vi "Wheel(2).vi"() -> ()   [LabVIEW 2020]
uses:
  <vilib>/DAQmx/read.llb/DAQmx Read (Counter DBL 1Chan 1Samp).vi
  <vilib>/DAQmx/create/channels.llb/DAQmx Create Channel (CI-Position-Angular Encoder).vi
  Shared/Experiment/ExperimentGlobals.vi
  <vilib>/Utility/file.llb/Write Delimited Spreadsheet (string).vi
  Shared/ModuleCrosstalk/Crosstalk.vi
  <vilib>/DAQmx/miscellaneous.llb/DAQmx Fill In Error Info.vi
  <vilib>/Utility/file.llb/Write Delimited Spreadsheet (DBL).vi
panel:
  out "Numeric":i32
  out "Speed av. 1s(cm/s) 2":dbl
  out "Output file":path
  out "Speed (cm/s)":dbl
  out "Counter task":refnum<k21>
  out "Aquiering":bool
  out "Distance (m)":dbl
  out "Angle (deg)":dbl
  out "Motion plot":dbl(graph)
  out "Recording":bool
  # "Mouse Wheel"
  # "Wires (left-right) : black-empty-green-orange-yellow"
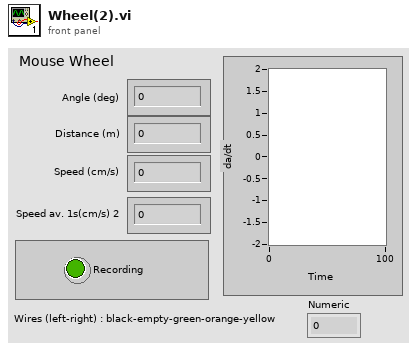
[diagram p1: front panel]
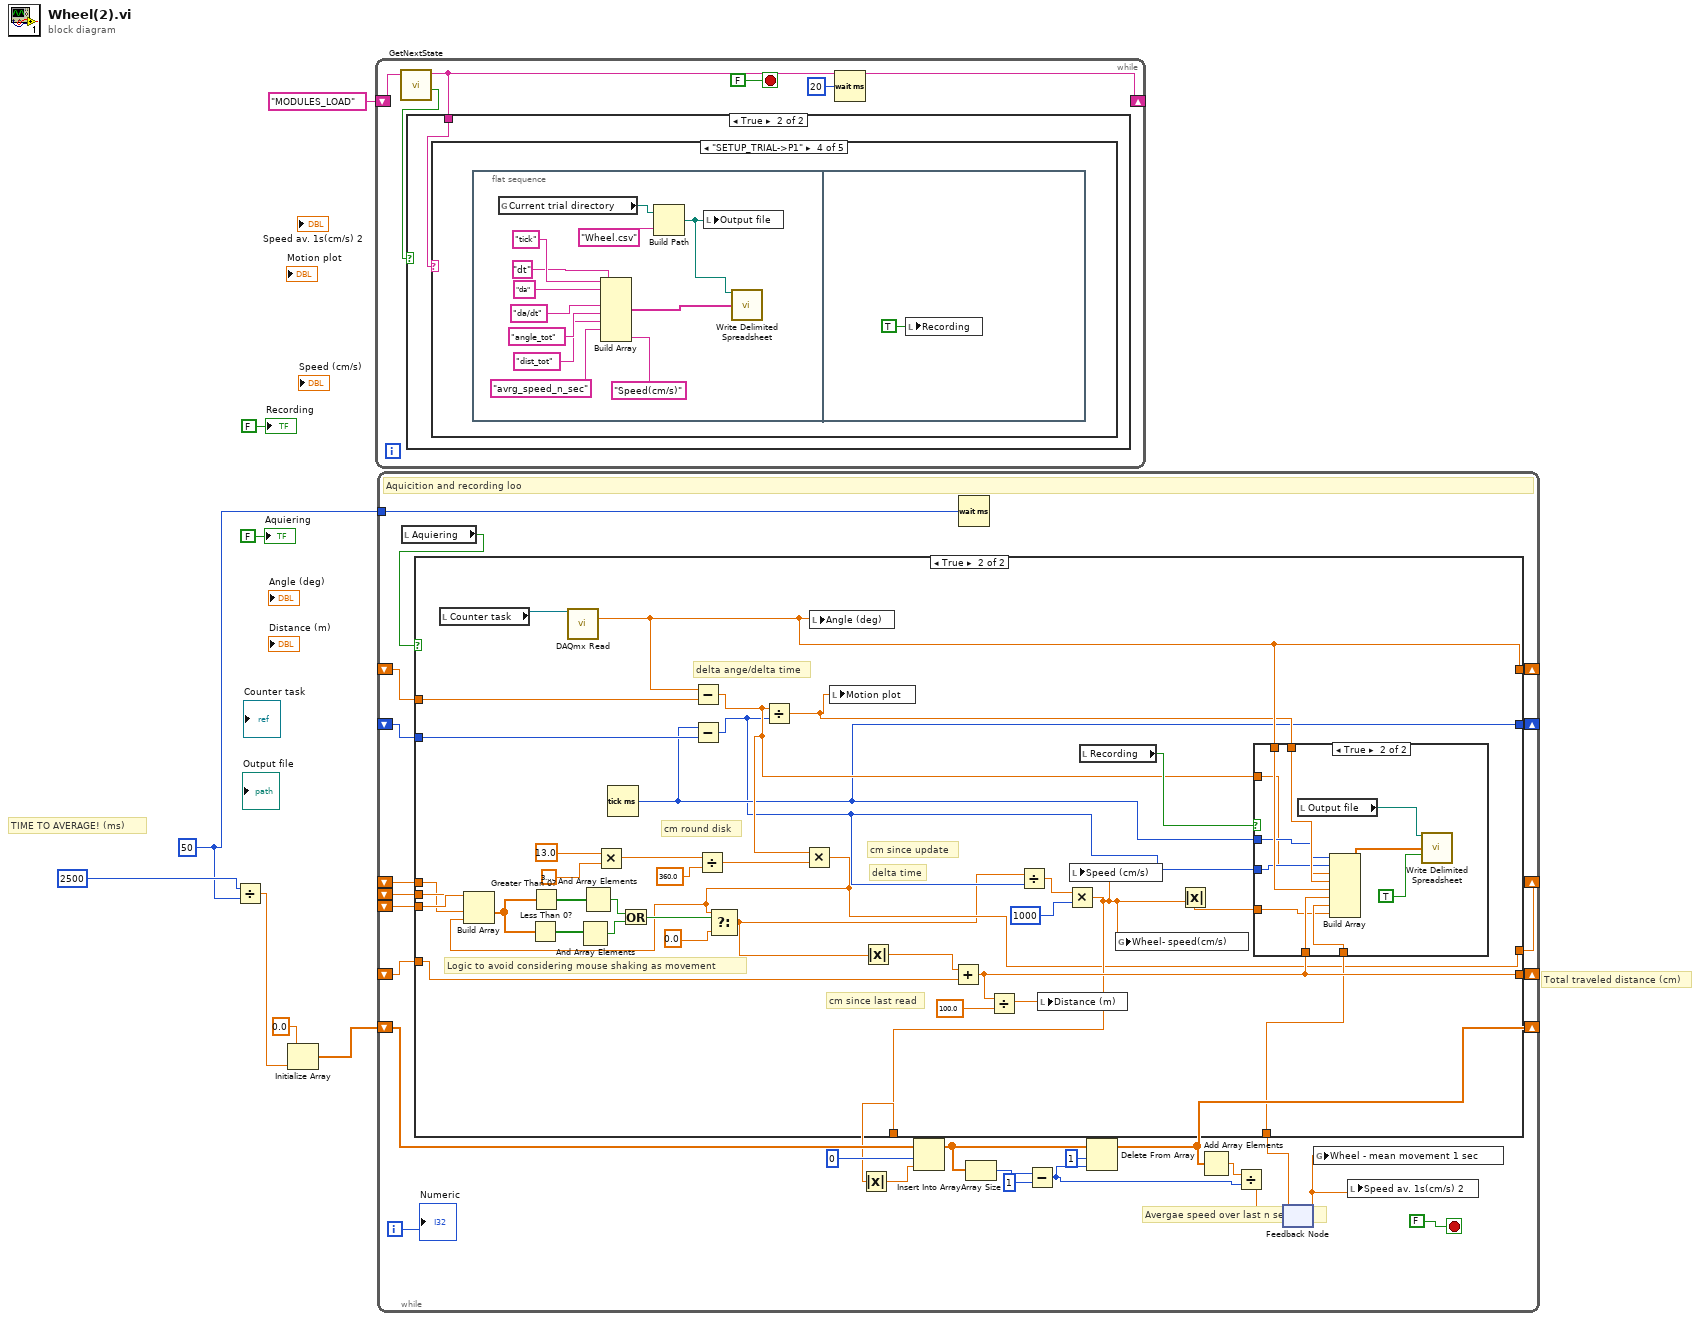
[diagram p0: block diagram]
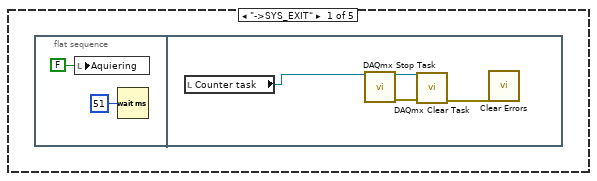
[diagram p5: hidden frame]
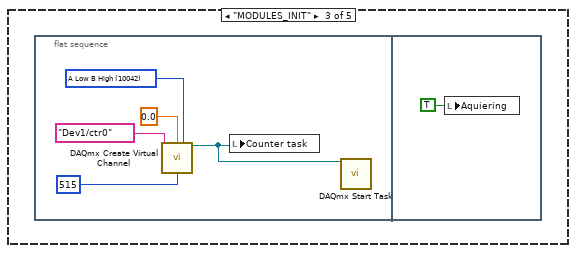
[diagram p7: hidden frame]
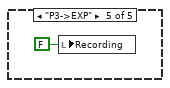
[diagram p8: hidden frame]
diagram:
  w4 = 50
  # "TIME TO AVERAGE! (ms)"
  # "Total traveled distance (cm)"
  n1 = Divide(x=2500, y=w4) -> (x/y=w3:dbl)
  n2 = Initialize Array(0.0, w3) -> (w1:dbl[])
  n3 = while {
    shift-right: [w9] -> _
    shift-left: "MODULES_LOAD" ("Next state") -> [w11]
    stop <- FALSE stop-if-true
    n4 = call "GetNextState.vi"("Current state"=w11) -> ("State has changed?"=w10:bool, "Next state"=w9:string)  [unwired: 9 in]
    n5 = case shown="True" w10 {
      tunnel: w9 -> [_ w14]
      frame False {
      }
      frame True {
        n6 = case shown="\"SETUP_TRIAL->P1\"" w14 {
          frame "->SYS_EXIT" {
            n7 = flat-sequence {
              frame #0 {
                n8 = local write "Aquiering"(FALSE ("Aquiering")) -> ()
                n9 = Wait (ms)(milliseconds to wait=u32 51) -> ()  [unwired: 1 out]
              }
              frame #1 {
                n10 = local read "Counter task"() -> (w17:refnum<k21>)
                n11 = call <vilib>:"DAQmx Stop Task.vi"("task/channels in"=w17) -> ("task out"=w18:refnum<k21>, "error out"=w19:errorcluster)  [unwired: 13 in]
                n12 = call <vilib>:"DAQmx Clear Task.vi"("task in"=w18, "error in"=w19) -> ("error out"=w20:errorcluster)  [unwired: 13 in]
                n13 = call <vilib>:"Clear Errors.vi"("error in (no error)"=w20) -> ()  [unwired: 5 in, 2 out]
              }
            }
          }
          frame Default {
          }
          frame "MODULES_INIT" {
            n14 = flat-sequence {
              frame #0 {
                w21 = 10042 items=["A High B High"=10040, "A High B Low"=10041, "A Low B High"=10042, "A Low B Low"=10043] ("z index phase")
                n15 = call-poly <vilib>:"DAQmx Create Virtual Channel.vi"("z index value"=0.0, "z index phase"=w21, "counter"=tag "Dev1/ctr0", "pulses per revolution"=u32 515) -> ("task out"=w23:refnum<k21>)  [unwired: 10 in, 1 out]
                n16 = local write "Counter task"(w23) -> ()
                n17 = call <vilib>:"DAQmx Start Task.vi"("task/channels in"=w23) -> ()  [unwired: 13 in, 2 out]
              }
              frame #1 {
                n18 = local write "Aquiering"(TRUE ("Aquiering")) -> ()
              }
            }
          }
          frame "SETUP_TRIAL->P1" {
            n19 = flat-sequence {
              frame #0 {
                n20 = global read "ExperimentGlobals.vi" "Current trial directory"() -> (w38:path)
                n21 = Build Array("tick", "dt" ("element"), "da" ("element"), "da/dt" ("element"), "angle_tot" ("element"), "dist_tot" ("element"), "avrg_speed_n_sec" ("element"), "Speed(cm/s)" ("element")) -> (w35:string[])
                n22 = Build Path(base path=w38, name or relative path="Wheel.csv") -> (appended path=w36:path)
                n23 = local write "Output file"(w36) -> ()
                n24 = call-poly <vilib>:"Write Delimited Spreadsheet.vi"("file path (dialog if empty)"=w36, "1D data"=w35) -> ()  [unwired: 12 in, 2 out]
              }
              frame #1 {
                n25 = local write "Recording"(TRUE ("Recording")) -> ()
              }
            }
          }
          frame "P3->EXP" {
            n26 = local write "Recording"(FALSE ("Recording")) -> ()
          }
        }
      }
    }
    n27 = Wait (ms)(milliseconds to wait=u32 20) -> ()  [unwired: 1 out]
  }
  n28 = while {
    shift-right: [w65] -> _
    shift-left: _ -> [w63]
    shift-right: [w64] -> _
    shift-left: _ -> [w62]
    shift-right: [w60] -> _
    shift-left: _ -> [w61]
    tunnel: w4 -> [w59]
    shift-right: [w51] -> _
    shift-left: w1 -> [w53]
    shift-right: [w44] -> _
    shift-left: _ -> [w41]
    shift-left: _ -> [w42]
    shift-left: _ -> [w43]
    i -> [w52]
    stop <- FALSE stop-if-true
    # "Avergae speed over last n seconds"
    # "Aquicition and recording loo"
    n29 = local read "Aquiering"() -> (w67:bool)
    n30 = Wait (ms)(milliseconds to wait=w59) -> ()  [unwired: 1 out]
    n31 = feedback #1() -> (w45:dbl)  [unwired: 1 in]
    n32 = case shown="True" w67 {
      tunnel: [_ w92] -> w65
      tunnel: [_ w88] -> w64
      tunnel: w63 -> [_ w102]
      tunnel: w62 -> [_ w101]
      tunnel: w61 -> [_ w98]
      tunnel: [_ w90] -> w60
      tunnel: [_ w85] -> w47
      tunnel: w45 -> [_ w86]
      tunnel: [_ w69] -> w44
      tunnel: w43 -> [_ w79]
      tunnel: w42 -> [_ w78]
      tunnel: w41 -> [_ w77]
      frame False {
      }
      frame True {
        # "Logic to avoid considering mouse shaking as movement"
        # "delta time"
        # "cm since update"
        # "delta ange/delta time"
        # "cm since last read"
        # "cm round disk"
        n33 = local read "Counter task"() -> (w103:refnum<k21>)
        n34 = call-poly <vilib>:"DAQmx Read.vi"("task/channels in"=w103) -> ("data"=w92:dbl)  [unwired: 12 in, 2 out]
        n35 = Multiply(x=13.0, y=3.141592653589793) -> (x*y=w81:dbl)
        n36 = Tick Count (ms)() -> (millisecond timer value=w88:u32)
        n37 = Subtract(x=w92, y=w102) -> (x-y=w89:dbl)
        n38 = Subtract(x=w88, y=w101) -> (x-y=w87:u32)
        n39 = Divide(x=w81, y=360.0) -> (x/y=w99:dbl)
        n40 = Divide(x=w89, y=w87) -> (x/y=w91:dbl)
        n41 = Multiply(x=w89, y=w99) -> (x*y=w69:dbl)
        n42 = Build Array(w79, w78, w77, w69) -> (w76:dbl[])
        n43 = Less Than 0?(x=w76) -> (x < 0?=w74:bool[])
        n44 = Greater Than 0?(x=w76) -> (x > 0?=w75:bool[])
        n45 = And Array Elements(Boolean array=w74) -> (logical AND=w73:bool)
        n46 = And Array Elements(Boolean array=w75) -> (logical AND=w72:bool)
        n47 = Or(x=w72, y=w73) -> (x .or. y?=w71:bool)
        n48 = Select(t=w69, s=w71, f=0.0) -> (s? t:f=w68:dbl)
        n49 = local write "Angle (deg)"(w92) -> ()
        n50 = local write "Motion plot"(w91) -> ()
        n51 = Absolute Value(x=w68) -> (abs(x)=w80:dbl)
        n52 = Add(x=w80, y=w98) -> (x+y=w90:dbl)
        n53 = Divide(x=w90, y=100.0) -> (x/y=w97:dbl)
        n54 = Divide(x=w68, y=w87) -> (x/y=w94:dbl)
        n55 = local write "Distance (m)"(w97) -> ()
        n56 = Multiply(x=w94, y=u32 1000) -> (x*y=w85:dbl)
        n57 = local write "Speed (cm/s)"(w85) -> ()
        n58 = local read "Recording"() -> (w93:bool)
        n59 = global write "Crosstalk.vi" "Wheel- speed(cm/s)"(w85) -> ()
        n60 = Absolute Value(x=w85) -> (abs(x)=w84:dbl)
        n61 = case shown="True" w93 {
          tunnel: w88 -> [_ w108]
          tunnel: w92 -> [_ w110]
          tunnel: w91 -> [_ w111]
          tunnel: w87 -> [_ w107]
          tunnel: w90 -> [_ w109]
          tunnel: w89 -> [_ w106]
          tunnel: w86 -> [_ w105]
          tunnel: w84 -> [_ w104]
          frame False {
          }
          frame True {
            n62 = local read "Output file"() -> (w114:path)
            n63 = Build Array(w108, w107, w106, w111, w110, w109, w105, w104) -> (w112:dbl[])
            n64 = call-poly <vilib>:"Write Delimited Spreadsheet.vi"("file path (dialog if empty)"=w114, "1D data"=w112, "append to file? (new file:F)"=TRUE ("append to file? (F)")) -> ()  [unwired: 11 in, 2 out]
          }
        }
      }
    }
    n65 = Absolute Value(x=w47) -> (abs(x)=w48:dbl)
    n66 = Insert Into Array(array=w53, index=0, new element=w48) -> (w55:dbl[])
    n67 = Array Size(array=w55) -> (size(s)=w56:i32)
    n68 = Subtract(x=w56, y=1) -> (x-y=w49:i32)
    n69 = Delete From Array(array=w55, length=1, index=w49) -> (array with subset deleted=w51:dbl[])  [unwired: 1 out]
    n70 = Add Array Elements(numeric array=w51) -> (sum=w50:dbl)
    n71 = Divide(x=w50, y=w49) -> (x/y=w46:dbl)
    n72 = feedback-in #1(w46) -> ()
    n73 = global write "Crosstalk.vi" "Wheel - mean movement 1 sec"(w45) -> ()
    n74 = local write "Speed av. 1s(cm/s) 2"(w45) -> ()
    "Numeric" <- w52
  }
  "Recording" <- FALSE ("Recording")
  "Aquiering" <- FALSE ("Aquiering")
